vi "SaveCardsIntoDB.vi"(8 "error in (no error)":errorcluster, 11 "ClashRoyale in":refnum<class "StashRoyale.lvclass">) -> (0 "error out":errorcluster, 3 "ClashRoyale out":refnum<class "StashRoyale.lvclass">)   [LabVIEW 2020, in "StashRoyale.lvclass"]
uses:
  StashRoyale.lvclass
  StashRoyale.lvclass/StashRoyale.ctl
  <vilib>/drjdpowell/SQLite Library/SQL Connection/Execute SQL (No results).vi
  <vilib>/drjdpowell/SQLite Library/SQLite.lvlib
  <vilib>/drjdpowell/SQLite Library/SQL Connection/Connection.lvclass
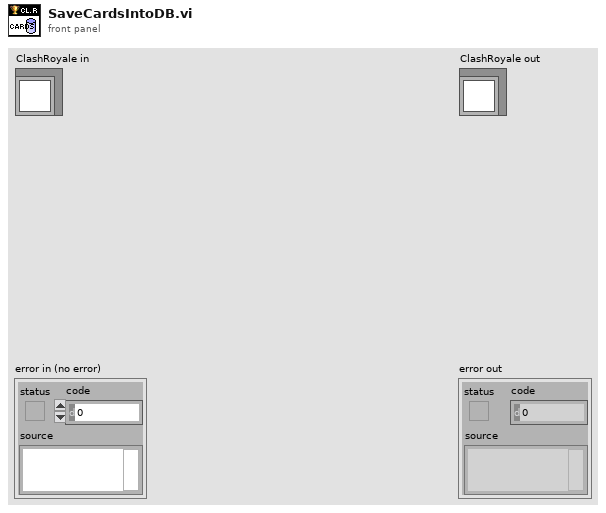
[diagram p1: front panel]
types:
  T1 = typedef "StashRoyale.lvclass/ctl_Card.ctl" = cluster{"name":string, "id":u32, "maxLevel":u8, "iconUrls":cluster{"medium":string}}
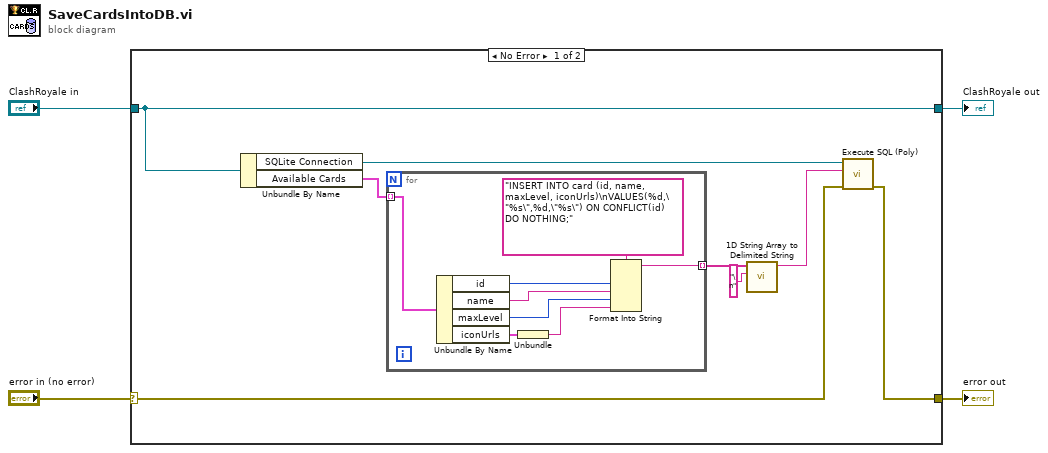
[diagram p0: block diagram]
diagram:
  n1 = case shown="No Error" "error in (no error)" {
    selector: "error in (no error)" -> [w9 w22]
    tunnel: [w11 w22] -> w3
    tunnel: [w10 w21] -> w1
    tunnel: "ClashRoyale in" -> [w10 w21]
    frame No Error {
      n2 = Unbundle By Name(w10) -> ("SQLite Connection"=w12:refnum<class "Connection.lvclass">, "Available Cards"=w8:T1[])
      n3 = for {
        tunnel: w8 -> [w18] mode=indexing
        tunnel: [w19] -> w7 mode=indexing
        n4 = Unbundle By Name(w18) -> ("id"=w17:u32, "name"=w16:string, "maxLevel"=w15:u8, "iconUrls"=w14:cluster{"medium":string})
        n5 = Unbundle(w14) -> ("medium"=w13:string)
        n6 = Format Into String(format string="INSERT INTO card (id, name, maxLevel, iconUrls)\nVALUES(%d,\"%s\",%d,\"%s\") ON CONFLICT(id) DO NOTHING;", w17, w16, w15, w13) -> (resulting string=w19:string)  [unwired: 2 in, 1 out]
      }
      n7 = call <vilib>:"1D String Array to Delimited String.vi"("delimiter"="\n", "string array"=w7) -> ("delimited string"=w6:string)  [unwired: 9 in]
      n8 = call-poly <vilib>:"Execute SQL (Poly).vi"("error in (no error)"=w9, "SQL"=w6, "SQLite Connection in"=w12) -> ("error out"=w11:errorcluster)  [unwired: 7 in, 1 out]
    }
    frame Error {
    }
  }
  "error out" <- w3
  "ClashRoyale out" <- w1
